vi "Periodic Tasks.vi"(8 "error in":errorcluster) -> ()   [LabVIEW 2013]
doc: "This VI runs in parallel to other tasks. It can contain as many user-defined periodic loops as you need. These can carry out PID or other sorts of timed response."
uses:
  Arm states.ctl
  tele shooter states.ctl
  <vilib>/Rock Robotics/SystemInterfaces/Utilities/FPGA_UtilitiesLED Source.ctl
  <vilib>/Rock Robotics/SystemInterfaces/Utilities/FPGA_UtilitiesLED State.ctl
  <vilib>/Rock Robotics/WPI/Relay/WPI_RelayValue.ctl
  Robot Global Data.vi
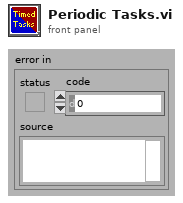
[diagram p1: front panel]
types:
  T1 = typedef "tele shooter states.ctl" = enum16{"button", "start", "stop"}
  T2 = typedef "Arm states.ctl" = enum16{"init", "frisbee", "left", "down", "close", "up", "right", "down 2", "open", "up 2"}
  T3 = typedef "WPI_MotorControlDeviceRef.ctl" = cluster{"DeviceStatus":errorcluster, "Type":enum16{"PWM", "CAN"}, "PWM":cluster{"Digital Module":T4, "PWM Channel":T5, "DeadBand":T6}, "CAN":cluster{"Device Number":u8, "Control Mode":T7, "Semaphore":T8, "Max Vout":dbl}, "Invert":bool, "TransformRef":T9, "InvTransformRef":T9}
  T4 = typedef "FPGA_TypedefDigitalModule.ctl" = enum16{"Digital Module 1", "Digital Module 2"}
  T5 = typedef "FPGA_DIOPWMChannel.ctl" = enum8{"PWM 1", "PWM 2", "PWM 3", "PWM 4", "PWM 5", "PWM 6", "PWM 7", "PWM 8", "PWM 9", "PWM 10", "Invalid"}
  T6 = typedef "WPI_PWMDeadband.ctl" = cluster{"Name":string, "maxPositivePwm":i32, "minPositivePwm":i32, "centerPwm":i32, "maxNegativePwm":i32, "minNegativePwm":i32, "angularRange":u16}
  T7 = typedef "WPI_CANJaguar_ControlMode.ctl" = enum8{"Percent VBus", "Current", "Speed", "Position", "Voltage"}
  T8 = typedef "Semaphore RefNum" = refnum<k1>
  T9 = typedef "WPI_PWMTransform_ConPane.ctl" = refnum<vi>
  T10 = typedef "WPI_DigitalInputDevRef.ctl" = cluster{"DevStatus":errorcluster, "DIO Channel":T11, "Digital Module":T4}
  T11 = typedef "FPGA_DIOChannel.ctl" = enum8{"DIO 1", "DIO 2", "DIO 3", "DIO 4", "DIO 5", "DIO 6", "DIO 7", "DIO 8", "DIO 9", "DIO 10", "DIO 11", "DIO 12", "DIO 13", "DIO 14", "Invalid"}
  T12 = typedef "WPI_RelayDevRef.ctl" = cluster{"DevStatus":errorcluster, "Relay Channel":T13, "Digital Module":T4, "Relay Direction":T14}
  T13 = typedef "FPGA_DIORelayChannel.ctl" = enum8{"Relay 1", "Relay 2", "Relay 3", "Relay 4", "Relay 5", "Relay 6", "Relay 7", "Relay 8", "Invalid"}
  T14 = typedef "WPI_RelayDirection.ctl" = enum16{"Both directions", "Forward only", "Reverse only"}
  T15 = typedef "FPGA_UtilitiesLED State.ctl" = enum16{"Off", "On", "Toggle"}
  T16 = typedef "FPGA_UtilitiesLED Source.ctl" = enum16{"User LED", "FPGA LED"}
  T17 = typedef "WPI_RelayValue.ctl" = enum16{"Off", "On", "Forward", "Reverse"}
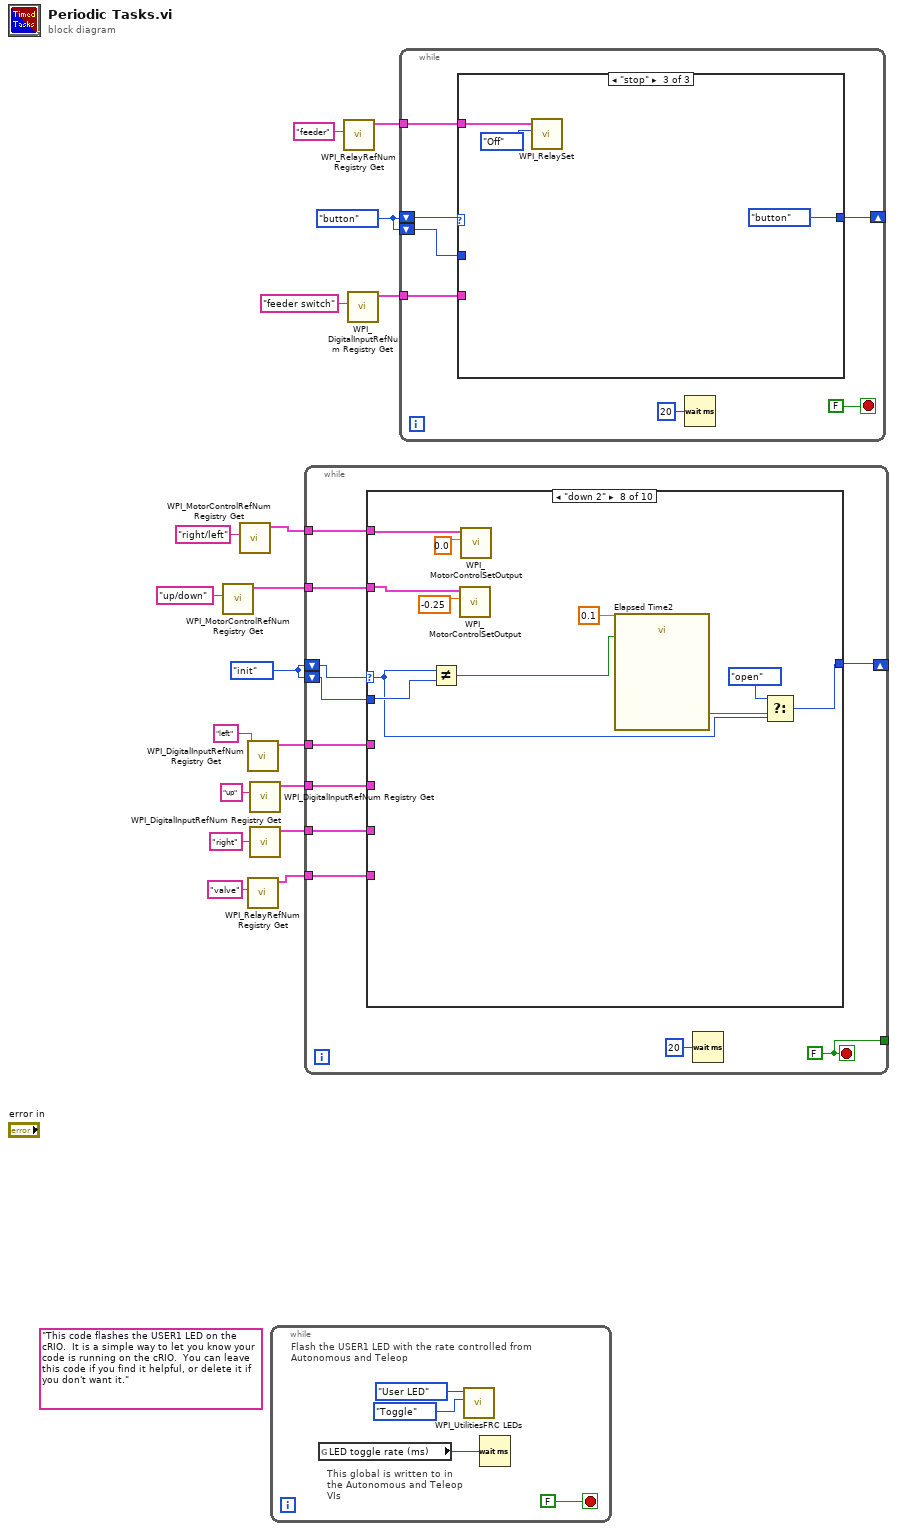
[diagram p0: block diagram]
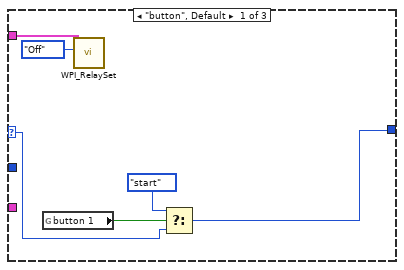
[diagram p2: hidden frame]
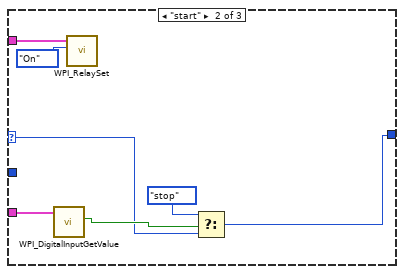
[diagram p3: hidden frame]
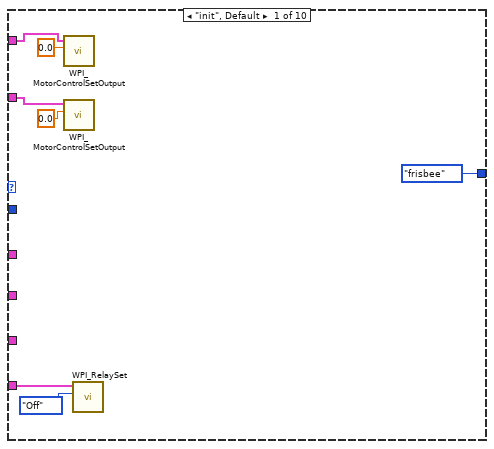
[diagram p4: hidden frame]
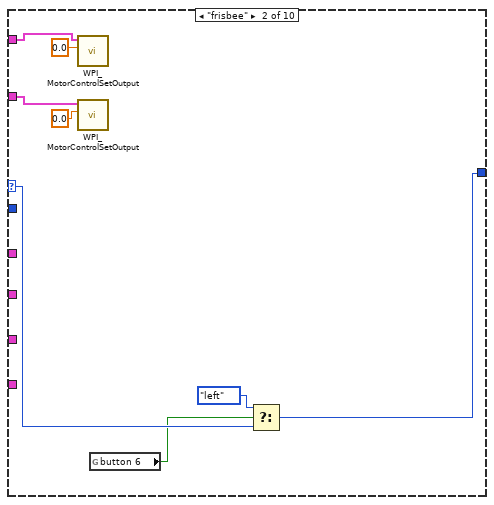
[diagram p5: hidden frame]
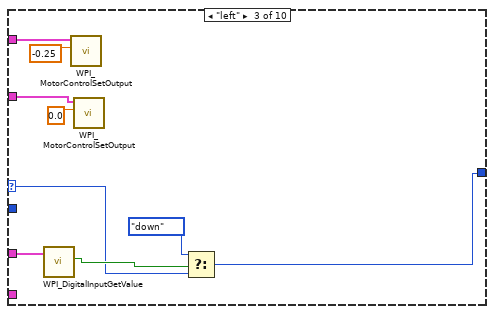
[diagram p6: hidden frame]
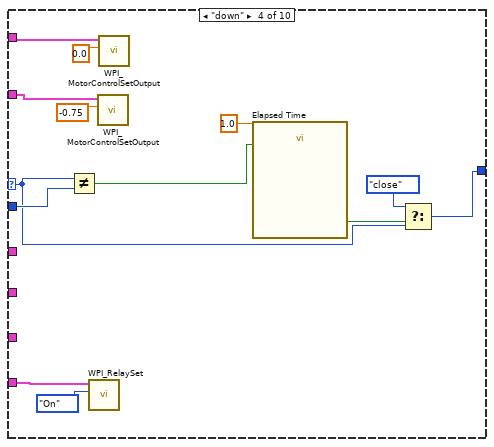
[diagram p7: hidden frame]
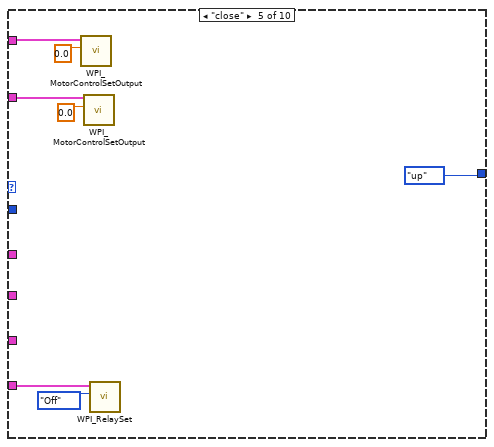
[diagram p8: hidden frame]
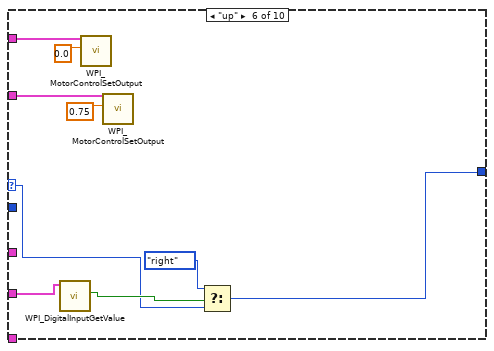
[diagram p9: hidden frame]
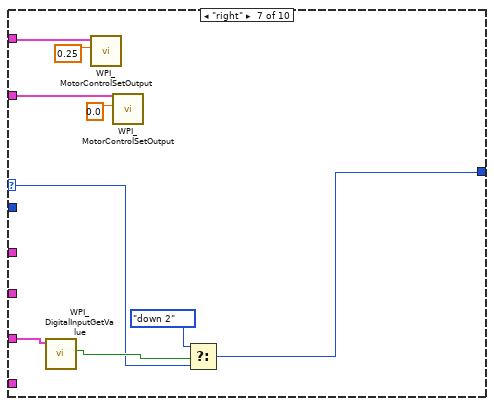
[diagram p10: hidden frame]
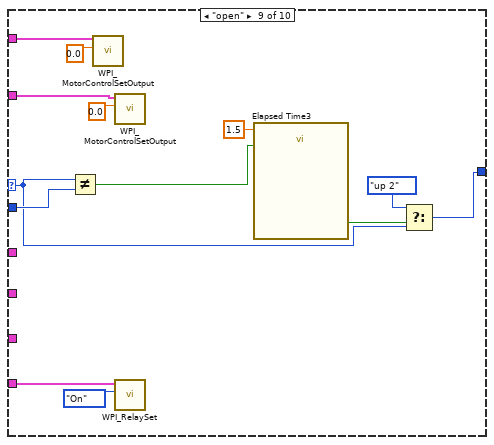
[diagram p11: hidden frame]
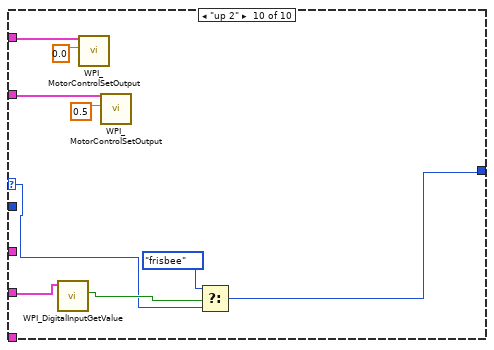
[diagram p12: hidden frame]
diagram:
  w5 = tele_shooter_states."button"
  w6 = Arm_states."init" ("Enum")
  (unwired) "This code flashes the USER1 LED on the cRIO.  It is a simple way to let you know your code is running on the cRIO.  You can leave this code if you find it helpful, or delete it if you don't want it."
  n1 = call <vilib>:"WPI_MotorControlRefNum Registry Get.vi"("refnum name"="up/down") -> ("MotorControlDevRef"=w17:T3)  [unwired: 9 in, 1 out]
  n2 = call <vilib>:"WPI_MotorControlRefNum Registry Get.vi"("refnum name"="right/left") -> ("MotorControlDevRef"=w18:T3)  [unwired: 9 in, 1 out]
  n3 = call <vilib>:"WPI_DigitalInputRefNum Registry Get.vi"("refnum name"="left") -> ("DigitalInputDevRef"=w11:T10)  [unwired: 9 in, 1 out]
  n4 = call <vilib>:"WPI_RelayRefNum Registry Get.vi"("refnum name"="valve") -> ("RelayDevRef"=w10:T12)  [unwired: 9 in, 1 out]
  n5 = call <vilib>:"WPI_DigitalInputRefNum Registry Get.vi"("refnum name"="up") -> ("DigitalInputDevRef"=w8:T10)  [unwired: 9 in, 1 out]
  n6 = call <vilib>:"WPI_DigitalInputRefNum Registry Get.vi"("refnum name"="right") -> ("DigitalInputDevRef"=w7:T10)  [unwired: 9 in, 1 out]
  n7 = while {
    stop <- FALSE stop-if-true
    # "This global is written to in the Autonomous and Teleop VIs"
    # "Flash the USER1 LED with the rate controlled from Autonomous and Teleop"
    n8 = global read "Robot Global Data.vi" "LED toggle rate (ms)"() -> (w19:u32)
    n9 = call <vilib>:"WPI_UtilitiesFRC LEDs.vi"("State"=FPGA_UtilitiesLED_State."Toggle", "LED Type"=FPGA_UtilitiesLED_Source."User LED") -> ()  [unwired: 1 in, 9 out]
    n10 = Wait (ms)(milliseconds to wait=w19) -> ()  [unwired: 1 out]
  }
  n11 = while {
    shift-right: [w31] -> _
    shift-left: w6 -> [w33]
    tunnel: [w32] -> _
    shift-left: w6 -> [w30]
    tunnel: w18 -> [w29]
    tunnel: w17 -> [w28]
    tunnel: w11 -> [w27]
    tunnel: w10 -> [w26]
    tunnel: w8 -> [w25]
    tunnel: w7 -> [w24]
    stop <- w32 stop-if-true
    w32 = FALSE
    n12 = case shown="\"down 2\"" w33 {
      selector: w33 -> [_ w44 w52 w63 _ w81 w90 w97 w108 w123]
      tunnel: [Arm_states."frisbee" ("Enum") w47 w55 w68 Arm_states."up" w83 w92 w96 w110 w120] -> w31
      tunnel: w30 -> [_ _ _ w64 _ _ _ w98 w109 _]
      tunnel: w29 -> [w36 w43 w51 w61 w73 w80 w89 w100 w116 w121]
      tunnel: w28 -> [w35 w42 w50 w60 w72 w79 w88 w99 w115 w122]
      tunnel: w27 -> [_ _ w49 _ _ _ _ _ _ _]
      tunnel: w26 -> [w34 _ _ w58 w71 _ _ _ w114 _]
      tunnel: w25 -> [_ _ _ _ _ w78 _ _ _ w124]
      tunnel: w24 -> [_ _ _ _ _ _ w87 _ _ _]
      frame "init", Default {
        n13 = call <vilib>:"WPI_MotorControlSetOutput.vi"("Output"=0.0, "MotorControlDevRef"=w36) -> ()  [unwired: 7 in, 3 out]
        n14 = call <vilib>:"WPI_MotorControlSetOutput.vi"("Output"=0.0, "MotorControlDevRef"=w35) -> ()  [unwired: 7 in, 3 out]
        n15 = call <vilib>:"WPI_RelaySet.vi"("RelayValue"=WPI_RelayValue."Off", "RelayDevRef"=w34) -> ()  [unwired: 8 in, 2 out]
      }
      frame "frisbee" {
        n16 = call <vilib>:"WPI_MotorControlSetOutput.vi"("Output"=0.0, "MotorControlDevRef"=w43) -> ()  [unwired: 7 in, 3 out]
        n17 = call <vilib>:"WPI_MotorControlSetOutput.vi"("Output"=0.0, "MotorControlDevRef"=w42) -> ()  [unwired: 7 in, 3 out]
        n18 = global read "Robot Global Data.vi" "button 6"() -> (w41:bool)
        n19 = Select(t=Arm_states."left", s=w41, f=w44) -> (s? t:f=w47:T2)
      }
      frame "left" {
        n20 = call <vilib>:"WPI_DigitalInputGetValue.vi"("DigitalInputDevRef"=w49) -> ("Value"=w53:bool)  [unwired: 8 in, 2 out]
        n21 = call <vilib>:"WPI_MotorControlSetOutput.vi"("Output"=-0.25, "MotorControlDevRef"=w51) -> ()  [unwired: 7 in, 3 out]
        n22 = call <vilib>:"WPI_MotorControlSetOutput.vi"("Output"=0.0, "MotorControlDevRef"=w50) -> ()  [unwired: 7 in, 3 out]
        n23 = Select(t=Arm_states."down", s=w53, f=w52) -> (s? t:f=w55:T2)
      }
      frame "down" {
        n24 = Not Equal?(x=w63, y=w64) -> (x != y?=w62:bool)
        n25 = call <vilib>:"WPI_RelaySet.vi"("RelayValue"=WPI_RelayValue."On", "RelayDevRef"=w58) -> ()  [unwired: 8 in, 2 out]
        n26 = call <vilib>:"WPI_MotorControlSetOutput.vi"("Output"=-0.75, "MotorControlDevRef"=w60) -> ()  [unwired: 7 in, 3 out]
        n27 = call <vilib>:"WPI_MotorControlSetOutput.vi"("Output"=0.0, "MotorControlDevRef"=w61) -> ()  [unwired: 7 in, 3 out]
        n28 = call "Elapsed Time"("Time Target (s)"=1.0, "Reset"=w62) -> ("Time has Elapsed"=w66:bool)  [unwired: 10 in, 7 out]
        n29 = Select(t=Arm_states."close", s=w66, f=w63) -> (s? t:f=w68:T2)
      }
      frame "close" {
        n30 = call <vilib>:"WPI_MotorControlSetOutput.vi"("Output"=0.0, "MotorControlDevRef"=w73) -> ()  [unwired: 7 in, 3 out]
        n31 = call <vilib>:"WPI_MotorControlSetOutput.vi"("Output"=0.0, "MotorControlDevRef"=w72) -> ()  [unwired: 7 in, 3 out]
        n32 = call <vilib>:"WPI_RelaySet.vi"("RelayValue"=WPI_RelayValue."Off", "RelayDevRef"=w71) -> ()  [unwired: 8 in, 2 out]
      }
      frame "up" {
        n33 = call <vilib>:"WPI_DigitalInputGetValue.vi"("DigitalInputDevRef"=w78) -> ("Value"=w82:bool)  [unwired: 8 in, 2 out]
        n34 = call <vilib>:"WPI_MotorControlSetOutput.vi"("Output"=0.0, "MotorControlDevRef"=w80) -> ()  [unwired: 7 in, 3 out]
        n35 = call <vilib>:"WPI_MotorControlSetOutput.vi"("Output"=0.75, "MotorControlDevRef"=w79) -> ()  [unwired: 7 in, 3 out]
        n36 = Select(t=Arm_states."right", s=w82, f=w81) -> (s? t:f=w83:T2)
      }
      frame "right" {
        n37 = call <vilib>:"WPI_DigitalInputGetValue.vi"("DigitalInputDevRef"=w87) -> ("Value"=w91:bool)  [unwired: 8 in, 2 out]
        n38 = call <vilib>:"WPI_MotorControlSetOutput.vi"("Output"=0.25, "MotorControlDevRef"=w89) -> ()  [unwired: 7 in, 3 out]
        n39 = call <vilib>:"WPI_MotorControlSetOutput.vi"("Output"=0.0, "MotorControlDevRef"=w88) -> ()  [unwired: 7 in, 3 out]
        n40 = Select(t=Arm_states."down 2", s=w91, f=w90) -> (s? t:f=w92:T2)
      }
      frame "down 2" {
        n41 = Not Equal?(x=w97, y=w98) -> (x != y?=w101:bool)
        n42 = call <vilib>:"WPI_MotorControlSetOutput.vi"("Output"=-0.25, "MotorControlDevRef"=w99) -> ()  [unwired: 7 in, 3 out]
        n43 = call <vilib>:"WPI_MotorControlSetOutput.vi"("Output"=0.0, "MotorControlDevRef"=w100) -> ()  [unwired: 7 in, 3 out]
        n44 = call "Elapsed Time2"("Time Target (s)"=0.1, "Reset"=w101) -> ("Time has Elapsed"=w103:bool)  [unwired: 10 in, 7 out]
        n45 = Select(t=Arm_states."open", s=w103, f=w97) -> (s? t:f=w96:T2)
      }
      frame "open" {
        n46 = Not Equal?(x=w108, y=w109) -> (x != y?=w111:bool)
        n47 = call <vilib>:"WPI_MotorControlSetOutput.vi"("Output"=0.0, "MotorControlDevRef"=w116) -> ()  [unwired: 7 in, 3 out]
        n48 = call <vilib>:"WPI_MotorControlSetOutput.vi"("Output"=0.0, "MotorControlDevRef"=w115) -> ()  [unwired: 7 in, 3 out]
        n49 = call <vilib>:"WPI_RelaySet.vi"("RelayValue"=WPI_RelayValue."On", "RelayDevRef"=w114) -> ()  [unwired: 8 in, 2 out]
        n50 = call "Elapsed Time3"("Time Target (s)"=1.5, "Reset"=w111) -> ("Time has Elapsed"=w112:bool)  [unwired: 10 in, 7 out]
        n51 = Select(t=Arm_states."up 2", s=w112, f=w108) -> (s? t:f=w110:T2)
      }
      frame "up 2" {
        n52 = call <vilib>:"WPI_DigitalInputGetValue.vi"("DigitalInputDevRef"=w124) -> ("Value"=w125:bool)  [unwired: 8 in, 2 out]
        n53 = call <vilib>:"WPI_MotorControlSetOutput.vi"("Output"=0.0, "MotorControlDevRef"=w121) -> ()  [unwired: 7 in, 3 out]
        n54 = call <vilib>:"WPI_MotorControlSetOutput.vi"("Output"=0.5, "MotorControlDevRef"=w122) -> ()  [unwired: 7 in, 3 out]
        n55 = Select(t=Arm_states."frisbee", s=w125, f=w123) -> (s? t:f=w120:T2)
      }
    }
    n56 = Wait (ms)(milliseconds to wait=u32 20) -> ()  [unwired: 1 out]
  }
  n57 = call <vilib>:"WPI_RelayRefNum Registry Get.vi"("refnum name"="feeder") -> ("RelayDevRef"=w3:T12)  [unwired: 9 in, 1 out]
  n58 = call <vilib>:"WPI_DigitalInputRefNum Registry Get.vi"("refnum name"="feeder switch") -> ("DigitalInputDevRef"=w1:T10)  [unwired: 9 in, 1 out]
  n59 = while {
    shift-right: [w133] -> _
    shift-left: w5 -> [w135]
    shift-left: w5 -> [w132]
    tunnel: w3 -> [w134]
    tunnel: w1 -> [w129]
    stop <- FALSE stop-if-true
    n60 = case shown="\"stop\"" w135 {
      selector: w135 -> [w137 w144 _]
      tunnel: w134 -> [w141 w148 w150]
      tunnel: [w138 w142 tele_shooter_states."button"] -> w133
      tunnel: w132 -> [_ _ _]
      tunnel: w129 -> [_ w145 _]
      frame "button", Default {
        n61 = global read "Robot Global Data.vi" "button 1"() -> (w139:bool)
        n62 = call <vilib>:"WPI_RelaySet.vi"("RelayValue"=WPI_RelayValue."Off", "RelayDevRef"=w141) -> ()  [unwired: 8 in, 2 out]
        n63 = Select(t=tele_shooter_states."start", s=w139, f=w137) -> (s? t:f=w138:T1)
      }
      frame "start" {
        n64 = call <vilib>:"WPI_DigitalInputGetValue.vi"("DigitalInputDevRef"=w145) -> ("Value"=w146:bool)  [unwired: 8 in, 2 out]
        n65 = call <vilib>:"WPI_RelaySet.vi"("RelayValue"=WPI_RelayValue."On", "RelayDevRef"=w148) -> ()  [unwired: 8 in, 2 out]
        n66 = Select(t=tele_shooter_states."stop", s=w146, f=w144) -> (s? t:f=w142:T1)
      }
      frame "stop" {
        n67 = call <vilib>:"WPI_RelaySet.vi"("RelayValue"=WPI_RelayValue."Off", "RelayDevRef"=w150) -> ()  [unwired: 8 in, 2 out]
      }
    }
    n68 = Wait (ms)(milliseconds to wait=u32 20) -> ()  [unwired: 1 out]
  }
